vi "DDS_Clock.vi"() -> ()   [LabVIEW 2016] (continued)
 "rel. amplitude CH1"=1.0, "phase [°] CH1"=0.0, "f0 [Hz] CH1"=310000000.0, "f1 [Hz] CH1"=310000000.0}, {"STEP"=0, "time[ms]"=0.05, "time tolerance[us]"=0.01, "CH0"=TRUE, "rel. amplitude CH0"=1.0, "phase [°] CH0"=0.0, "f0 [Hz] CH0"=313000000.0, "f1 [Hz] CH0"=313200000.00000006, "CH1"=FALSE, "rel. amplitude CH1"=1.0, "phase [°] CH1"=0.0, "f0 [Hz] CH1"=310000000.0, "f1 [Hz] CH1"=310000000.0}, {"STEP"=0, "time[ms]"=0.05, "time tolerance[us]"=0.01, "CH0"=TRUE, "rel. amplitude CH0"=1.0, "phase [°] CH0"=0.0, "f0 [Hz] CH0"=313200000.00000006, "f1 [Hz] CH0"=313400000.00000006, "CH1"=FALSE, "rel. amplitude CH1"=1.0, "phase [°] CH1"=0.0, "f0 [Hz] CH1"=310000000.0, "f1 [Hz] CH1"=310000000.0}, {"STEP"=0, "time[ms]"=0.05, "time tolerance[us]"=0.01, "CH0"=TRUE, "rel. amplitude CH0"=1.0, "phase [°] CH0"=0.0, "f0 [Hz] CH0"=313400000.00000006, "f1 [Hz] CH0"=313600000.0, "CH1"=FALSE, "rel. amplitude CH1"=1.0, "phase [°] CH1"=0.0, "f0 [Hz] CH1"=310000000.0, "f1 [Hz] CH1"=310000000.0}, {"STEP"=0, "time[ms]"=0.05, "time tolerance[us]"=0.01, "CH0"=TRUE, "rel. amplitude CH0"=1.0, "phase [°] CH0"=0.0, "f0 [Hz] CH0"=313600000.0, "f1 [Hz] CH0"=313800000.0, "CH1"=FALSE, "rel. amplitude CH1"=1.0, "phase [°] CH1"=0.0, "f0 [Hz] CH1"=310000000.0, "f1 [Hz] CH1"=310000000.0}, {"STEP"=0, "time[ms]"=0.05, "time tolerance[us]"=0.01, "CH0"=TRUE, "rel. amplitude CH0"=1.0, "phase [°] CH0"=0.0, "f0 [Hz] CH0"=313800000.0, "f1 [Hz] CH0"=314000000.0, "CH1"=FALSE, "rel. amplitude CH1"=1.0, "phase [°] CH1"=0.0, "f0 [Hz] CH1"=310000000.0, "f1 [Hz] CH1"=310000000.0}, {"STEP"=0, "time[ms]"=0.05, "time tolerance[us]"=0.01, "CH0"=TRUE, "rel. amplitude CH0"=1.0, "phase [°] CH0"=0.0, "f0 [Hz] CH0"=314000000.0, "f1 [Hz] CH0"=314200000.0, "CH1"=FALSE, "rel. amplitude CH1"=1.0, "phase [°] CH1"=0.0, "f0 [Hz] CH1"=310000000.0, "f1 [Hz] CH1"=310000000.0}, {"STEP"=0, "time[ms]"=0.05, "time tolerance[us]"=0.01, "CH0"=TRUE, "rel. amplitude CH0"=1.0, "phase [°] CH0"=0.0, "f0 [Hz] CH0"=314200000.0, "f1 [Hz] CH0"=314400000.0, "CH1"=FALSE, "rel. amplitude CH1"=1.0, "phase [°] CH1"=0.0, "f0 [Hz] CH1"=310000000.0, "f1 [Hz] CH1"=310000000.0}, {"STEP"=0, "time[ms]"=0.05, "time tolerance[us]"=0.01, "CH0"=TRUE, "rel. amplitude CH0"=1.0, "phase [°] CH0"=0.0, "f0 [Hz] CH0"=314400000.0, "f1 [Hz] CH0"=314600000.00000006, "CH1"=FALSE, "rel. amplitude CH1"=1.0, "phase [°] CH1"=0.0, "f0 [Hz] CH1"=310000000.0, "f1 [Hz] CH1"=310000000.0}, {"STEP"=0, "time[ms]"=0.05, "time tolerance[us]"=0.01, "CH0"=TRUE, "rel. amplitude CH0"=1.0, "phase [°] CH0"=0.0, "f0 [Hz] CH0"=314600000.00000006, "f1 [Hz] CH0"=314800000.00000006, "CH1"=FALSE, "rel. amplitude CH1"=1.0, "phase [°] CH1"=0.0, "f0 [Hz] CH1"=310000000.0, "f1 [Hz] CH1"=310000000.0}, {"STEP"=0, "time[ms]"=0.05, "time tolerance[us]"=0.01, "CH0"=TRUE, "rel. amplitude CH0"=1.0, "phase [°] CH0"=0.0, "f0 [Hz] CH0"=314800000.00000006, "f1 [Hz] CH0"=315000000.0, "CH1"=FALSE, "rel. amplitude CH1"=1.0, "phase [°] CH1"=0.0, "f0 [Hz] CH1"=310000000.0, "f1 [Hz] CH1"=310000000.0}, {"STEP"=0, "time[ms]"=0.05, "time tolerance[us]"=0.01, "CH0"=TRUE, "rel. amplitude CH0"=1.0, "phase [°] CH0"=0.0, "f0 [Hz] CH0"=315000000.0, "f1 [Hz] CH0"=315200000.00000006, "CH1"=FALSE, "rel. amplitude CH1"=1.0, "phase [°] CH1"=0.0, "f0 [Hz] CH1"=310000000.0, "f1 [Hz] CH1"=310000000.0}, {"STEP"=0, "time[ms]"=0.05, "time tolerance[us]"=0.01, "CH0"=TRUE, "rel. amplitude CH0"=1.0, "phase [°] CH0"=0.0, "f0 [Hz] CH0"=315200000.00000006, "f1 [Hz] CH0"=315400000.0, "CH1"=FALSE, "rel. amplitude CH1"=1.0, "phase [°] CH1"=0.0, "f0 [Hz] CH1"=310000000.0, "f1 [Hz] CH1"=310000000.0}, {"STEP"=0, "time[ms]"=0.05, "time tolerance[us]"=0.01, "CH0"=TRUE, "rel. amplitude CH0"=1.0, "phase [°] CH0"=0.0, "f0 [Hz] CH0"=315400000.0, "f1 [Hz] CH0"=315600000.0, "CH1"=FALSE, "rel. amplitude CH1"=1.0, "phase [°] CH1"=0.0, "f0 [Hz] CH1"=310000000.0, "f1 [Hz] CH1"=310000000.0}, {"STEP"=0, "time[ms]"=0.05, "time tolerance[us]"=0.01, "CH0"=TRUE, "rel. amplitude CH0"=1.0, "phase [°] CH0"=0.0, "f0 [Hz] CH0"=315600000.0, "f1 [Hz] CH0"=315800000.0, "CH1"=FALSE, "rel. amplitude CH1"=1.0, "phase [°] CH1"=0.0, "f0 [Hz] CH1"=310000000.0, "f1 [Hz] CH1"=310000000.0}, {"STEP"=0, "time[ms]"=0.05, "time tolerance[us]"=0.01, "CH0"=TRUE, "rel. amplitude CH0"=1.0, "phase [°] CH0"=0.0, "f0 [Hz] CH0"=315800000.0, "f1 [Hz] CH0"=316000000.0, "CH1"=FALSE, "rel. amplitude CH1"=1.0, "phase [°] CH1"=0.0, "f0 [Hz] CH1"=310000000.0, "f1 [Hz] CH1"=310000000.0}, {"STEP"=0, "time[ms]"=0.05, "time tolerance[us]"=0.01, "CH0"=TRUE, "rel. amplitude CH0"=1.0, "phase [°] CH0"=0.0, "f0 [Hz] CH0"=316000000.0, "f1 [Hz] CH0"=316200000.0, "CH1"=FALSE, "rel. amplitude CH1"=1.0, "phase [°] CH1"=0.0, "f0 [Hz] CH1"=310000000.0, "f1 [Hz] CH1"=310000000.0}, {"STEP"=0, "time[ms]"=0.05, "time tolerance[us]"=0.01, "CH0"=TRUE, "rel. amplitude CH0"=1.0, "phase [°] CH0"=0.0, "f0 [Hz] CH0"=316200000.0, "f1 [Hz] CH0"=316400000.00000006, "CH1"=FALSE, "rel. amplitude CH1"=1.0, "phase [°] CH1"=0.0, "f0 [Hz] CH1"=310000000.0, "f1 [Hz] CH1"=310000000.0}, {"STEP"=0, "time[ms]"=0.05, "time tolerance[us]"=0.01, "CH0"=TRUE, "rel. amplitude CH0"=1.0, "phase [°] CH0"=0.0, "f0 [Hz] CH0"=316400000.00000006, "f1 [Hz] CH0"=316600000.00000006, "CH1"=FALSE, "rel. amplitude CH1"=1.0, "phase [°] CH1"=0.0, "f0 [Hz] CH1"=310000000.0, "f1 [Hz] CH1"=310000000.0}, {"STEP"=0, "time[ms]"=0.05, "time tolerance[us]"=0.01, "CH0"=TRUE, "rel. amplitude CH0"=1.0, "phase [°] CH0"=0.0, "f0 [Hz] CH0"=316600000.00000006, "f1 [Hz] CH0"=316800000.00000006, "CH1"=FALSE, "rel. amplitude CH1"=1.0, "phase [°] CH1"=0.0, "f0 [Hz] CH1"=310000000.0, "f1 [Hz] CH1"=310000000.0}, {"STEP"=0, "time[ms]"=0.05, "time tolerance[us]"=0.01, "CH0"=TRUE, "rel. amplitude CH0"=1.0, "phase [°] CH0"=0.0, "f0 [Hz] CH0"=316800000.00000006, "f1 [Hz] CH0"=317000000.0, "CH1"=FALSE, "rel. amplitude CH1"=1.0, "phase [°] CH1"=0.0, "f0 [Hz] CH1"=310000000.0, "f1 [Hz] CH1"=310000000.0}, {"STEP"=0, "time[ms]"=0.05, "time tolerance[us]"=0.01, "CH0"=TRUE, "rel. amplitude CH0"=1.0, "phase [°] CH0"=0.0, "f0 [Hz] CH0"=317000000.0, "f1 [Hz] CH0"=317200000.0, "CH1"=FALSE, "rel. amplitude CH1"=1.0, "phase [°] CH1"=0.0, "f0 [Hz] CH1"=310000000.0, "f1 [Hz] CH1"=310000000.0}, {"STEP"=0, "time[ms]"=0.05, "time tolerance[us]"=0.01, "CH0"=TRUE, "rel. amplitude CH0"=1.0, "phase [°] CH0"=0.0, "f0 [Hz] CH0"=317200000.0, "f1 [Hz] CH0"=317400000.00000006, "CH1"=FALSE, "rel. amplitude CH1"=1.0, "phase [°] CH1"=0.0, "f0 [Hz] CH1"=310000000.0, "f1 [Hz] CH1"=310000000.0}, {"STEP"=0, "time[ms]"=0.05, "time tolerance[us]"=0.01, "CH0"=TRUE, "rel. amplitude CH0"=1.0, "phase [°] CH0"=0.0, "f0 [Hz] CH0"=317400000.00000006, "f1 [Hz] CH0"=317600000.00000006, "CH1"=FALSE, "rel. amplitude CH1"=1.0, "phase [°] CH1"=0.0, "f0 [Hz] CH1"=310000000.0, "f1 [Hz] CH1"=310000000.0}, {"STEP"=0, "time[ms]"=0.05, "time tolerance[us]"=0.01, "CH0"=TRUE, "rel. amplitude CH0"=1.0, "phase [°] CH0"=0.0, "f0 [Hz] CH0"=317600000.00000006, "f1 [Hz] CH0"=317800000.0, "CH1"=FALSE, "rel. amplitude CH1"=1.0, "phase [°] CH1"=0.0, "f0 [Hz] CH1"=310000000.0, "f1 [Hz] CH1"=310000000.0}, {"STEP"=0, "time[ms]"=0.05, "time tolerance[us]"=0.01, "CH0"=TRUE, "rel. amplitude CH0"=1.0, "phase [°] CH0"=0.0, "f0 [Hz] CH0"=317800000.0, "f1 [Hz] CH0"=318000000.0, "CH1"=FALSE, "rel. amplitude CH1"=1.0, "phase [°] CH1"=0.0, "f0 [Hz] CH1"=310000000.0, "f1 [Hz] CH1"=310000000.0}, {"STEP"=0, "time[ms]"=0.05, "time tolerance[us]"=0.01, "CH0"=TRUE, "rel. amplitude CH0"=1.0, "phase [°] CH0"=0.0, "f0 [Hz] CH0"=318000000.0, "f1 [Hz] CH0"=318200000.0, "CH1"=FALSE, "rel. amplitude CH1"=1.0, "phase [°] CH1"=0.0, "f0 [Hz] CH1"=310000000.0, "f1 [Hz] CH1"=310000000.0}, {"STEP"=0, "time[ms]"=0.05, "time tolerance[us]"=0.01, "CH0"=TRUE, "rel. amplitude CH0"=1.0, "phase [°] CH0"=0.0, "f0 [Hz] CH0"=318200000.0, "f1 [Hz] CH0"=318400000.00000006, "CH1"=FALSE, "rel. amplitude CH1"=1.0, "phase [°] CH1"=0.0, "f0 [Hz] CH1"=310000000.0, "f1 [Hz] CH1"=310000000.0}, {"STEP"=0, "time[ms]"=0.05, "time tolerance[us]"=0.01, "CH0"=TRUE, "rel. amplitude CH0"=1.0, "phase [°] CH0"=0.0, "f0 [Hz] CH0"=318400000.00000006, "f1 [Hz] CH0"=318600000.0, "CH1"=FALSE, "rel. amplitude CH1"=1.0, "phase [°] CH1"=0.0, "f0 [Hz] CH1"=310000000.0, "f1 [Hz] CH1"=310000000.0}, {"STEP"=0, "time[ms]"=0.05, "time tolerance[us]"=0.01, "CH0"=TRUE, "rel. amplitude CH0"=1.0, "phase [°] CH0"=0.0, "f0 [Hz] CH0"=318600000.0, "f1 [Hz] CH0"=318800000.0, "CH1"=FALSE, "rel. amplitude CH1"=1.0, "phase [°] CH1"=0.0, "f0 [Hz] CH1"=310000000.0, "f1 [Hz] CH1"=310000000.0}, {"STEP"=0, "time[ms]"=0.05, "time tolerance[us]"=0.01, "CH0"=TRUE, "rel. amplitude CH0"=1.0, "phase [°] CH0"=0.0, "f0 [Hz] CH0"=318800000.0, "f1 [Hz] CH0"=319000000.0, "CH1"=FALSE, "rel. amplitude CH1"=1.0, "phase [°] CH1"=0.0, "f0 [Hz] CH1"=310000000.0, "f1 [Hz] CH1"=310000000.0}, {"STEP"=0, "time[ms]"=0.05, "time tolerance[us]"=0.01, "CH0"=TRUE, "rel. amplitude CH0"=1.0, "phase [°] CH0"=0.0, "f0 [Hz] CH0"=319000000.0, "f1 [Hz] CH0"=319200000.0, "CH1"=FALSE, "rel. amplitude CH1"=1.0, "phase [°] CH1"=0.0, "f0 [Hz] CH1"=310000000.0, "f1 [Hz] CH1"=310000000.0}, {"STEP"=0, "time[ms]"=0.05, "time tolerance[us]"=0.01, "CH0"=TRUE, "rel. amplitude CH0"=1.0, "phase [°] CH0"=0.0, "f0 [Hz] CH0"=319200000.0, "f1 [Hz] CH0"=319400000.00000006, "CH1"=FALSE, "rel. amplitude CH1"=1.0, "phase [°] CH1"=0.0, "f0 [Hz] CH1"=310000000.0, "f1 [Hz] CH1"=310000000.0}, {"STEP"=0, "time[ms]"=0.05, "time tolerance[us]"=0.01, "CH0"=TRUE, "rel. amplitude CH0"=1.0, "phase [°] CH0"=0.0, "f0 [Hz] CH0"=319400000.00000006, "f1 [Hz] CH0"=319600000.00000006, "CH1"=FALSE, "rel. amplitude CH1"=1.0, "phase [°] CH1"=0.0, "f0 [Hz] CH1"=310000000.0, "f1 [Hz] CH1"=310000000.0}, {"STEP"=0, "time[ms]"=0.05, "time tolerance[us]"=0.01, "CH0"=TRUE, "rel. amplitude CH0"=1.0, "phase [°] CH0"=0.0, "f0 [Hz] CH0"=319600000.00000006, "f1 [Hz] CH0"=319800000.00000006, "CH1"=FALSE, "rel. amplitude CH1"=1.0, "phase [°] CH1"=0.0, "f0 [Hz] CH1"=310000000.0, "f1 [Hz] CH1"=310000000.0}, {"STEP"=0, "time[ms]"=0.05, "time tolerance[us]"=0.01, "CH0"=TRUE, "rel. amplitude CH0"=1.0, "phase [°] CH0"=0.0, "f0 [Hz] CH0"=319800000.00000006, "f1 [Hz] CH0"=320000000.0, "CH1"=FALSE, "rel. amplitude CH1"=1.0, "phase [°] CH1"=0.0, "f0 [Hz] CH1"=310000000.0, "f1 [Hz] CH1"=310000000.0}, {"STEP"=0, "time[ms]"=0.05, "time tolerance[us]"=0.01, "CH0"=TRUE, "rel. amplitude CH0"=1.0, "phase [°] CH0"=0.0, "f0 [Hz] CH0"=320000000.0, "f1 [Hz] CH0"=319800000.0, "CH1"=FALSE, "rel. amplitude CH1"=1.0, "phase [°] CH1"=0.0, "f0 [Hz] CH1"=310000000.0, "f1 [Hz] CH1"=310000000.0}, {"STEP"=0, "time[ms]"=0.05, "time tolerance[us]"=0.01, "CH0"=TRUE, "rel. amplitude CH0"=1.0, "phase [°] CH0"=0.0, "f0 [Hz] CH0"=319800000.0, "f1 [Hz] CH0"=319599999.99999994, "CH1"=FALSE, "rel. amplitude CH1"=1.0, "phase [°] CH1"=0.0, "f0 [Hz] CH1"=310000000.0, "f1 [Hz] CH1"=310000000.0}, {"STEP"=0, "time[ms]"=0.05, "time tolerance[us]"=0.01, "CH0"=TRUE, "rel. amplitude CH0"=1.0, "phase [°] CH0"=0.0, "f0 [Hz] CH0"=319599999.99999994, "f1 [Hz] CH0"=319400000.0, "CH1"=FALSE, "rel. amplitude CH1"=1.0, "phase [°] CH1"=0.0, "f0 [Hz] CH1"=310000000.0, "f1 [Hz] CH1"=310000000.0}, {"STEP"=0, "time[ms]"=0.05, "time tolerance[us]"=0.01, "CH0"=TRUE, "rel. amplitude CH0"=1.0, "phase [°] CH0"=0.0, "f0 [Hz] CH0"=319400000.0, "f1 [Hz] CH0"=319200000.0, "CH1"=FALSE, "rel. amplitude CH1"=1.0, "phase [°] CH1"=0.0, "f0 [Hz] CH1"=310000000.0, "f1 [Hz] CH1"=310000000.0}, {"STEP"=0, "time[ms]"=0.05, "time tolerance[us]"=0.01, "CH0"=TRUE, "rel. amplitude CH0"=1.0, "phase [°] CH0"=0.0, "f0 [Hz] CH0"=319200000.0, "f1 [Hz] CH0"=319000000.0, "CH1"=FALSE, "rel. amplitude CH1"=1.0, "phase [°] CH1"=0.0, "f0 [Hz] CH1"=310000000.0, "f1 [Hz] CH1"=310000000.0}, {"STEP"=0, "time[ms]"=0.05, "time tolerance[us]"=0.01, "CH0"=TRUE, "rel. amplitude CH0"=1.0, "phase [°] CH0"=0.0, "f0 [Hz] CH0"=319000000.0, "f1 [Hz] CH0"=318800000.0, "CH1"=FALSE, "rel. amplitude CH1"=1.0, "phase [°] CH1"=0.0, "f0 [Hz] CH1"=310000000.0, "f1 [Hz] CH1"=310000000.0}, {"STEP"=0, "time[ms]"=0.05, "time tolerance[us]"=0.01, "CH0"=TRUE, "rel. amplitude CH0"=1.0, "phase [°] CH0"=0.0, "f0 [Hz] CH0"=318800000.0, "f1 [Hz] CH0"=318599999.99999994, "CH1"=FALSE, "rel. amplitude CH1"=1.0, "phase [°] CH1"=0.0, "f0 [Hz] CH1"=310000000.0, "f1 [Hz] CH1"=310000000.0}, {"STEP"=0, "time[ms]"=0.05, "time tolerance[us]"=0.01, "CH0"=TRUE, "rel. amplitude CH0"=1.0, "phase [°] CH0"=0.0, "f0 [Hz] CH0"=318599999.99999994, "f1 [Hz] CH0"=318399999.99999994, "CH1"=FALSE, "rel. amplitude CH1"=1.0, "phase [°] CH1"=0.0, "f0 [Hz] CH1"=310000000.0, "f1 [Hz] CH1"=310000000.0}, {"STEP"=0, "time[ms]"=0.05, "time tolerance[us]"=0.01, "CH0"=TRUE, "rel. amplitude CH0"=1.0, "phase [°] CH0"=0.0, "f0 [Hz] CH0"=318399999.99999994, "f1 [Hz] CH0"=318199999.99999994, "CH1"=FALSE, "rel. amplitude CH1"=1.0, "phase [°] CH1"=0.0, "f0 [Hz] CH1"=310000000.0, "f1 [Hz] CH1"=310000000.0}, {"STEP"=0, "time[ms]"=0.05, "time tolerance[us]"=0.01, "CH0"=TRUE, "rel. amplitude CH0"=1.0, "phase [°] CH0"=0.0, "f0 [Hz] CH0"=318199999.99999994, "f1 [Hz] CH0"=318000000.0, "CH1"=FALSE, "rel. amplitude CH1"=1.0, "phase [°] CH1"=0.0, "f0 [Hz] CH1"=310000000.0, "f1 [Hz] CH1"=310000000.0}, {"STEP"=0, "time[ms]"=0.05, "time tolerance[us]"=0.01, "CH0"=TRUE, "rel. amplitude CH0"=1.0, "phase [°] CH0"=0.0, "f0 [Hz] CH0"=318000000.0, "f1 [Hz] CH0"=317800000.0, "CH1"=FALSE, "rel. amplitude CH1"=1.0, "phase [°] CH1"=0.0, "f0 [Hz] CH1"=310000000.0, "f1 [Hz] CH1"=310000000.0}, {"STEP"=0, "time[ms]"=0.05, "time tolerance[us]"=0.01, "CH0"=TRUE, "rel. amplitude CH0"=1.0, "phase [°] CH0"=0.0, "f0 [Hz] CH0"=317800000.0, "f1 [Hz] CH0"=317599999.99999994, "CH1"=FALSE, "rel. amplitude CH1"=1.0, "phase [°] CH1"=0.0, "f0 [Hz] CH1"=310000000.0, "f1 [Hz] CH1"=310000000.0}, {"STEP"=0, "time[ms]"=0.05, "time tolerance[us]"=0.01, "CH0"=TRUE, "rel. amplitude CH0"=1.0, "phase [°] CH0"=0.0, "f0 [Hz] CH0"=317599999.99999994, "f1 [Hz] CH0"=317399999.99999994, "CH1"=FALSE, "rel. amplitude CH1"=1.0, "phase [°] CH1"=0.0, "f0 [Hz] CH1"=310000000.0, "f1 [Hz] CH1"=310000000.0}, {"STEP"=0, "time[ms]"=0.05, "time tolerance[us]"=0.01, "CH0"=TRUE, "rel. amplitude CH0"=1.0, "phase [°] CH0"=0.0, "f0 [Hz] CH0"=317399999.99999994, "f1 [Hz] CH0"=317200000.0, "CH1"=FALSE, "rel. amplitude CH1"=1.0, "phase [°] CH1"=0.0, "f0 [Hz] CH1"=310000000.0, "f1 [Hz] CH1"=310000000.0}, {"STEP"=0, "time[ms]"=0.05, "time tolerance[us]"=0.01, "CH0"=TRUE, "rel. amplitude CH0"=1.0, "phase [°] CH0"=0.0, "f0 [Hz] CH0"=317200000.0, "f1 [Hz] CH0"=317000000.0, "CH1"=FALSE, "rel. amplitude CH1"=1.0, "phase [°] CH1"=0.0, "f0 [Hz] CH1"=310000000.0, "f1 [Hz] CH1"=310000000.0}, {"STEP"=0, "time[ms]"=0.05, "time tolerance[us]"=0.01, "CH0"=TRUE, "rel. amplitude CH0"=1.0, "phase [°] CH0"=0.0, "f0 [Hz] CH0"=317000000.0, "f1 [Hz] CH0"=316800000.0, "CH1"=FALSE, "rel. amplitude CH1"=1.0, "phase [°] CH1"=0.0, "f0 [Hz] CH1"=310000000.0, "f1 [Hz] CH1"=310000000.0}, {"STEP"=0, "time[ms]"=0.05, "time tolerance[us]"=0.01, "CH0"=TRUE, "rel. amplitude CH0"=1.0, "phase [°] CH0"=0.0, "f0 [Hz] CH0"=316800000.0, "f1 [Hz] CH0"=316599999.99999994, "CH1"=FALSE, "rel. amplitude CH1"=1.0, "phase [°] CH1"=0.0, "f0 [Hz] CH1"=310000000.0, "f1 [Hz] CH1"=310000000.0}, {"STEP"=0, "time[ms]"=0.05, "time tolerance[us]"=0.01, "CH0"=TRUE, "rel. amplitude CH0"=1.0, "phase [°] CH0"=0.0, "f0 [Hz] CH0"=316599999.99999994, "f1 [Hz] CH0"=316400000.0, "CH1"=FALSE, "rel. amplitude CH1"=1.0, "phase [°] CH1"=0.0, "f0 [Hz] CH1"=310000000.0, "f1 [Hz] CH1"=310000000.0}, {"STEP"=0, "time[ms]"=0.05, "time tolerance[us]"=0.01, "CH0"=TRUE, "rel. amplitude CH0"=1.0, "phase [°] CH0"=0.0, "f0 [Hz] CH0"=316400000.0, "f1 [Hz] CH0"=316200000.0, "CH1"=FALSE, "rel. amplitude CH1"=1.0, "phase [°] CH1"=0.0, "f0 [Hz] CH1"=310000000.0, "f1 [Hz] CH1"=310000000.0}, {"STEP"=0, "time[ms]"=0.05, "time tolerance[us]"=0.01, "CH0"=TRUE, "rel. amplitude CH0"=1.0, "phase [°] CH0"=0.0, "f0 [Hz] CH0"=316200000.0, "f1 [Hz] CH0"=316000000.0, "CH1"=FALSE, "rel. amplitude CH1"=1.0, "phase [°] CH1"=0.0, "f0 [Hz] CH1"=310000000.0, "f1 [Hz] CH1"=310000000.0}, {"STEP"=0, "time[ms]"=0.05, "time tolerance[us]"=0.01, "CH0"=TRUE, "rel. amplitude CH0"=1.0, "phase [°] CH0"=0.0, "f0 [Hz] CH0"=316000000.0, "f1 [Hz] CH0"=315800000.0, "CH1"=FALSE, "rel. amplitude CH1"=1.0, "phase [°] CH1"=0.0, "f0 [Hz] CH1"=310000000.0, "f1 [Hz] CH1"=310000000.0}, {"STEP"=0, "time[ms]"=0.05, "time tolerance[us]"=0.01, "CH0"=TRUE, "rel. amplitude CH0"=1.0, "phase [°] CH0"=0.0, "f0 [Hz] CH0"=315800000.0, "f1 [Hz] CH0"=315599999.99999994, "CH1"=FALSE, "rel. amplitude CH1"=1.0, "phase [°] CH1"=0.0, "f0 [Hz] CH1"=310000000.0, "f1 [Hz] CH1"=310000000.0}, {"STEP"=0, "time[ms]"=0.05, "time tolerance[us]"=0.01, "CH0"=TRUE, "rel. amplitude CH0"=1.0, "phase [°] CH0"=0.0, "f0 [Hz] CH0"=315599999.99999994, "f1 [Hz] CH0"=315399999.99999994, "CH1"=FALSE, "rel. amplitude CH1"=1.0, "phase [°] CH1"=0.0, "f0 [Hz] CH1"=310000000.0, "f1 [Hz] CH1"=310000000.0}, {"STEP"=0, "time[ms]"=0.05, "time tolerance[us]"=0.01, "CH0"=TRUE, "rel. amplitude CH0"=1.0, "phase [°] CH0"=0.0, "f0 [Hz] CH0"=315399999.99999994, "f1 [Hz] CH0"=315199999.99999994, "CH1"=FALSE, "rel. amplitude CH1"=1.0, "phase [°] CH1"=0.0, "f0 [Hz] CH1"=310000000.0, "f1 [Hz] CH1"=310000000.0}, {"STEP"=0, "time[ms]"=0.05, "time tolerance[us]"=0.01, "CH0"=TRUE, "rel. amplitude CH0"=1.0, "phase [°] CH0"=0.0, "f0 [Hz] CH0"=315199999.99999994, "f1 [Hz] CH0"=315000000.0, "CH1"=FALSE, "rel. amplitude CH1"=1.0, "phase [°] CH1"=0.0, "f0 [Hz] CH1"=310000000.0, "f1 [Hz] CH1"=310000000.0}, {"STEP"=0, "time[ms]"=0.05, "time tolerance[us]"=0.01, "CH0"=TRUE, "rel. amplitude CH0"=1.0, "phase [°] CH0"=0.0, "f0 [Hz] CH0"=315000000.0, "f1 [Hz] CH0"=314800000.0, "CH1"=FALSE, "rel. amplitude CH1"=1.0, "phase [°] CH1"=0.0, "f0 [Hz] CH1"=310000000.0, "f1 [Hz] CH1"=310000000.0}, {"STEP"=0, "time[ms]"=0.05, "time tolerance[us]"=0.01, "CH0"=TRUE, "rel. amplitude CH0"=1.0, "phase [°] CH0"=0.0, "f0 [Hz] CH0"=314800000.0, "f1 [Hz] CH0"=314599999.99999994, "CH1"=FALSE, "rel. amplitude CH1"=1.0, "phase [°] CH1"=0.0, "f0 [Hz] CH1"=310000000.0, "f1 [Hz] CH1"=310000000.0}, {"STEP"=0, "time[ms]"=0.05, "time tolerance[us]"=0.01, "CH0"=TRUE, "rel. amplitude CH0"=1.0, "phase [°] CH0"=0.0, "f0 [Hz] CH0"=314599999.99999994, "f1 [Hz] CH0"=314400000.0, "CH1"=FALSE, "rel. amplitude CH1"=1.0, "phase [°] CH1"=0.0, "f0 [Hz] CH1"=310000000.0, "f1 [Hz] CH1"=310000000.0}, {"STEP"=0, "time[ms]"=0.05, "time tolerance[us]"=0.01, "CH0"=TRUE, "rel. amplitude CH0"=1.0, "phase [°] CH0"=0.0, "f0 [Hz] CH0"=314400000.0, "f1 [Hz] CH0"=314200000.0, "CH1"=FALSE, "rel. amplitude CH1"=1.0, "phase [°] CH1"=0.0, "f0 [Hz] CH1"=310000000.0, "f1 [Hz] CH1"=310000000.0}, {"STEP"=0, "time[ms]"=0.05, "time tolerance[us]"=0.01, "CH0"=TRUE, "rel. amplitude CH0"=1.0, "phase [°] CH0"=0.0, "f0 [Hz] CH0"=314200000.0, "f1 [Hz] CH0"=314000000.0, "CH1"=FALSE, "rel. amplitude CH1"=1.0, "phase [°] CH1"=0.0, "f0 [Hz] CH1"=310000000.0, "f1 [Hz] CH1"=310000000.0}, {"STEP"=0, "time[ms]"=0.05, "time tolerance[us]"=0.01, "CH0"=TRUE, "rel. amplitude CH0"=1.0, "phase [°] CH0"=0.0, "f0 [Hz] CH0"=314000000.0, "f1 [Hz] CH0"=313800000.0, "CH1"=FALSE, "rel. amplitude CH1"=1.0, "phase [°] CH1"=0.0, "f0 [Hz] CH1"=310000000.0, "f1 [Hz] CH1"=310000000.0}, {"STEP"=0, "time[ms]"=0.05, "time tolerance[us]"=0.01, "CH0"=TRUE, "rel. amplitude CH0"=1.0, "phase [°] CH0"=0.0, "f0 [Hz] CH0"=313800000.0, "f1 [Hz] CH0"=313599999.99999994, "CH1"=FALSE, "rel. amplitude CH1"=1.0, "phase [°] CH1"=0.0, "f0 [Hz] CH1"=310000000.0, "f1 [Hz] CH1"=310000000.0}, {"STEP"=0, "time[ms]"=0.05, "time tolerance[us]"=0.01, "CH0"=TRUE, "rel. amplitude CH0"=1.0, "phase [°] CH0"=0.0, "f0 [Hz] CH0"=313599999.99999994, "f1 [Hz] CH0"=313399999.99999994, "CH1"=FALSE, "rel. amplitude CH1"=1.0, "phase [°] CH1"=0.0, "f0 [Hz] CH1"=310000000.0, "f1 [Hz] CH1"=310000000.0}, {"STEP"=0, "time[ms]"=0.05, "time tolerance[us]"=0.01, "CH0"=TRUE, "rel. amplitude CH0"=1.0, "phase [°] CH0"=0.0, "f0 [Hz] CH0"=313399999.99999994, "f1 [Hz] CH0"=313199999.99999994, "CH1"=FALSE, "rel. amplitude CH1"=1.0, "phase [°] CH1"=0.0, "f0 [Hz] CH1"=310000000.0, "f1 [Hz] CH1"=310000000.0}, 
